vi "Motor-Controls.vi"(6 "Downwards":i16, 7 "Still":i16, 8 "Upwards":i16) -> ()   [LabVIEW 2020]
uses:
  <userlib>/_NI I2C IP/FPGA/Public/I2C Interface.ctl
  <userlib>/_NI I2C IP/FPGA/Public/Data Array Type.ctl
  <userlib>/_NI I2C IP/FPGA/Public/Word Controller Settings.ctl
  <vilib>/rvi/Emulation/niFpgaGetClockAttributes.vi
  <vilib>/rvi/Emulation/niFpgaSctlEmulationGetInTimedLoop.vi
  <vilib>/rvi/Emulation/niFpgaEmulationReportErrorSimple.vi
  <vilib>/rvi/Emulation/niFpgaCriticalErrorInLSC.vi
  <userlib>/_NI I2C IP/FPGA/NI I2C IP FPGA.lvlib
panel:
  in  "settings":T1
  in  "write data":T2=[0, 0, 0, 0, 0, 0, 0, 0] format="%.0x"
  in  "go":bool
  in  "direction ready":bool
  in  "i2c bus in":T3
  out "ready for input":bool
  out "read data":T2 format="%.0x"
  out "i2c bus out":T3
  out "Downwards 2":i16
  out "Still 2":i16
  out "Upwards 2":i16
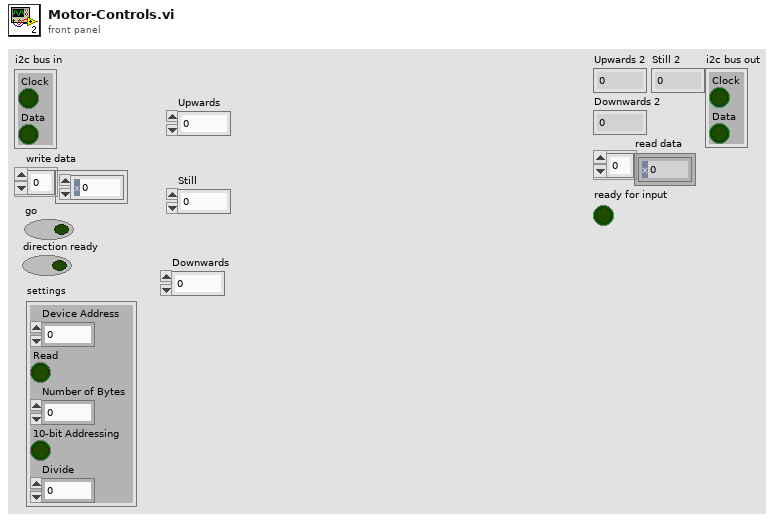
[diagram p1: front panel]
types:
  T1 = typedef "NI I2C IP FPGA.lvlib/Word Controller Settings.ctl" = cluster{"Device Address":u16, "Read":bool, "Number of Bytes":u8, "10-bit Addressing":bool, "Divide":u8}
  T2 = typedef "NI I2C IP FPGA.lvlib/Data Array Type.ctl" = u8[]
  T3 = typedef "NI I2C IP FPGA.lvlib/I2C Interface.ctl" = cluster{"Clock":bool, "Data":bool}
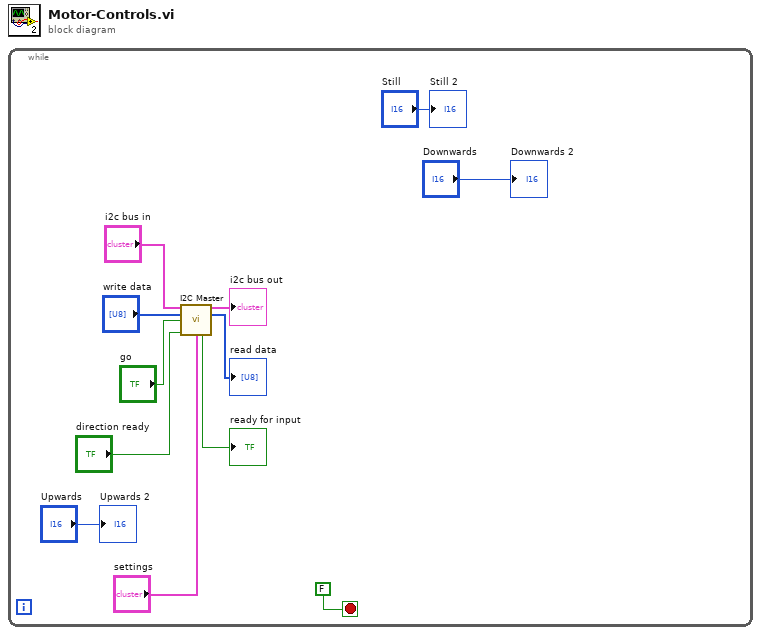
[diagram p0: block diagram]
diagram:
  n1 = while {
    stop <- FALSE stop-if-true
    n2 = call <userlib>:"I2C Master.vi"("i2c bus in"="i2c bus in", "write data"="write data", "go"="go", "direction ready"="direction ready", "settings"="settings") -> ("i2c bus out"=→"i2c bus out":T3, "read data"=→"read data":T2, "ready for input"=→"ready for input":bool)  [unwired: 8 in]
    "Upwards 2" <- "Upwards"
    "Still 2" <- "Still"
    "Downwards 2" <- "Downwards"
  }
